vi "Next.vi"(8 "Error In":errorcluster, 11 "Reader In":refnum<class "String.lvclass">) -> (0 "Error Out":errorcluster, 1 "Done":bool, 2 "Character":u8, 3 "Reader Out":refnum<class "String.lvclass">)   [LabVIEW 2018, in "Toolkit.lvlib" / "Readers.lvlib" / "String.lvclass"]
uses:
  String.lvclass
  String.lvclass/String.ctl
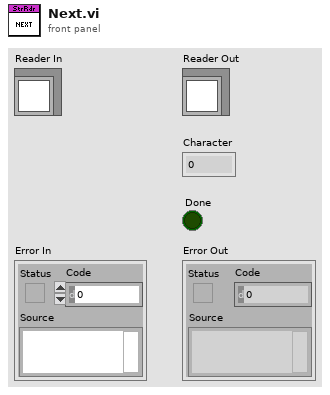
[diagram p1: front panel]
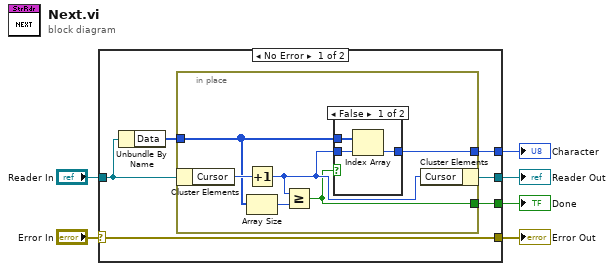
[diagram p0: block diagram]
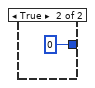
[diagram p2: hidden frame]
diagram:
  n1 = case shown="No Error" "Error In" {
    selector: "Error In" -> [w8 w24]
    tunnel: [w8 w24] -> w5
    tunnel: "Reader In" -> [w12 w23]
    tunnel: [w10 w23] -> w3
    tunnel: [w9 _] -> w2
    tunnel: [w7 _] -> w1
    frame No Error {
      n2 = Unbundle By Name(w12) -> ("Data"=w11:u8[])
      n3 = in-place {
        in-place-border: w11 -> [w16]
        in-place-border: [w14] -> w9
        in-place-border: [w13] -> w7
        n4 = in-place-cluster #1(w12) -> ("Cursor"=w18:i32)
        n5 = Increment(x=w18) -> (x+1=w15:i32)
        n6 = Array Size(array=w16) -> (size(s)=w17:i32)
        n7 = Greater Or Equal?(x=w15, y=w17) -> (x >= y?=w13:bool)
        n8 = case shown="False" w13 {
          tunnel: w16 -> [w21 _]
          tunnel: w15 -> [w20 _]
          tunnel: [w19 u8 0 ("Character")] -> w14
          frame False {
            n9 = Index Array(array=w21, index=w20) -> (element=w19:u8)
          }
          frame True {
          }
        }
        n10 = in-place-cluster #1("Cursor"=w15) -> (w10:refnum<class "String.lvclass">)
      }
    }
    frame Error {
    }
  }
  "Error Out" <- w5
  "Reader Out" <- w3
  "Character" <- w2
  "Done" <- w1
